vi "log.vi"(8 "error in (no error)":errorcluster, 10 "log_entry":T1 {"datetime" format="%<%x %.3X>T"}, 11 "system.logging.provider in":refnum<class "system.logging.provider.lvclass">) -> (0 "error out":errorcluster, 3 "system.logging.provider out":refnum<class "system.logging.provider.lvclass">)   [LabVIEW 2021, in "system.logging.provider.lvclass"]
uses:
  system.logging.provider.lvclass
  system.logging/log_entry.ctl
  system.logging/severity.ctl
  system.logging.provider.lvclass/system.logging.provider.ctl
  system.logging/system.logging.lvclass
panel:
  out "log_entry_display":T1 {"datetime" format="%<%x %.3X>T"}
  # "Entry will be displayed if provider criteria is met.\n\nThis is just an example, this VI should be overriden\nfor the specific provider implementation."
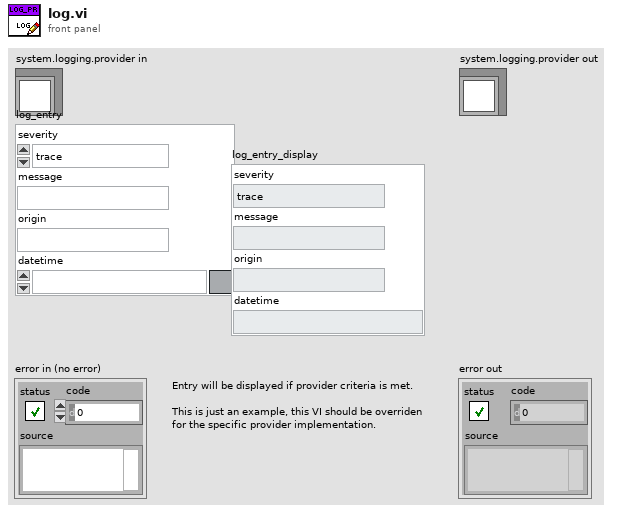
[diagram p1: front panel]
types:
  T1 = typedef "system.logging.lvclass/log_entry.ctl" = cluster{"severity":T2, "message":string, "origin":string, "datetime":timestamp}
  T2 = typedef "system.logging.lvclass/severity.ctl" = enum8{"trace", "debug", "info", "warning", "error"}
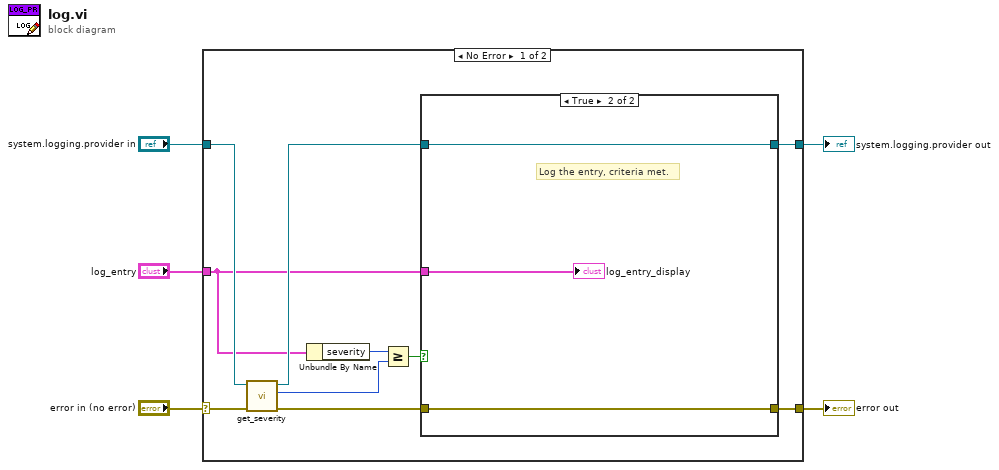
[diagram p0: block diagram]
diagram:
  n1 = case shown="No Error" "error in (no error)" {
    selector: "error in (no error)" -> [w15 w22]
    tunnel: [w8 w22] -> w4
    tunnel: [w7 w21] -> w2
    tunnel: "system.logging.provider in" -> [w14 w21]
    tunnel: "log_entry" -> [w6 _]
    frame No Error {
      n2 = call "get_severity.vi"("error in (no error)"=w15, "system.logging.provider in"=w14) -> ("error out"=w10:errorcluster, "severity"=w12:T2, "system.logging.provider out"=w9:refnum<class "system.logging.provider.lvclass">)  [unwired: 7 in]
      n3 = Unbundle By Name(w6) -> ("severity"=w13:T2)
      n4 = Greater Or Equal?(x=w13, y=w12) -> (x >= y?=w11:bool)
      n5 = case shown="True" w11 {
        tunnel: w10 -> [w17 w19]
        tunnel: w9 -> [w16 w20]
        tunnel: [w17 w19] -> w8
        tunnel: [w16 w20] -> w7
        tunnel: w6 -> [_ w18]
        frame False {
          # "Discard, entry"
        }
        frame True {
          # "Log the entry, criteria met."
          "log_entry_display" <- w18
        }
      }
    }
    frame Error {
    }
  }
  "error out" <- w4
  "system.logging.provider out" <- w2
